vi "Test DAQ IO API.vi"() -> ()   [LabVIEW 2016]
doc: "DAQ IO API Tester."
uses:
  DI Channel Setting.ctl
  DO Channel Setting.ctl
  <vilib>/Utility/miscctls.llb/LVPointTypeDef.ctl
  <vilib>/Utility/error.llb/DialogType.ctl
  DAQ IO.lvlib
panel:
  in  "REQ Retry DI":bool
  in  "REQ Wakeup_helper_loop_DI":bool
  in  "DO Channel Setting":T1
  in  "REQ Acq DI":bool
  in  "DI Channel Setting":T2
  out "Acquire DI":bool[](array[boolean])
  in  "REQ Close DO":bool
  in  "REQ Close DI":bool
  in  "DO Value":bool[](array[boolean])
  in  "REQ Write DO":bool
  out "Connect?":bool
  out "Connect?":bool
  in  "REQ Initialize DO":bool
  in  "DAQ Type":enum16{"Hardware", "Simulation"}(ring)
  in  "REQ Initialize DI":bool
  in  "Show Diagram on Init":bool
  in  "Show Block Diagram":bool
  in  "Stop Module":bool
  in  "Start Module":bool
  in  "Hide Module Panel":bool
  in  "Show Module Panel":bool
  out "Status":string
  out "Module Running?":bool
  # "This VI tests the API for the Module."
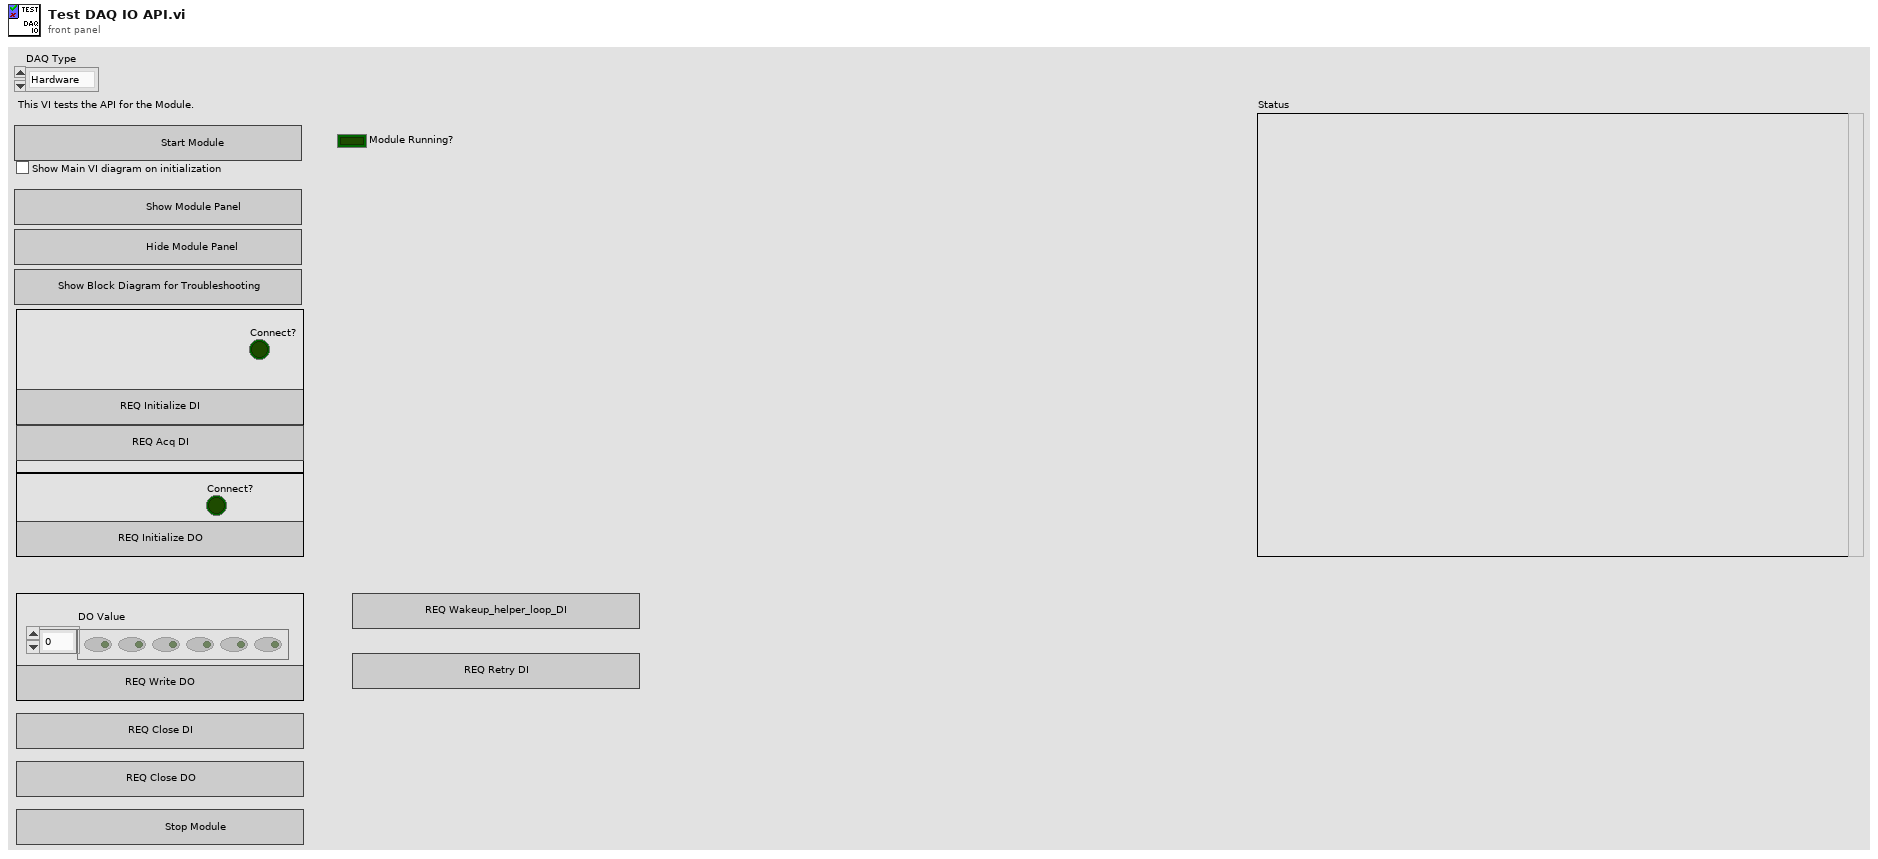
[diagram p1: front panel]
types:
  T1 = typedef "DAQ IO.lvlib/DO Channel Setting.ctl" = cluster{"DO Channel":string[]}
  T2 = typedef "DAQ IO.lvlib/DI Channel Setting.ctl" = cluster{"Channel":string[]}
  T3 = typedef "LVPointTypeDef.ctl" = cluster{"Horizontal":i16, "Vertical":i16}
  T4 = typedef "DAQ IO.lvlib/Broadcast Events--cluster.ctl" = cluster{"Module Did Init":refnum<user-event>, "Status Updated":refnum<user-event>, "Error Reported":refnum<user-event>, "Module Did Stop":refnum<user-event>, "Update Module Execution Status":refnum<user-event>, "REQ Broadcast DI":refnum<user-event>}
  T5 = typedef "DialogType.ctl" = u16
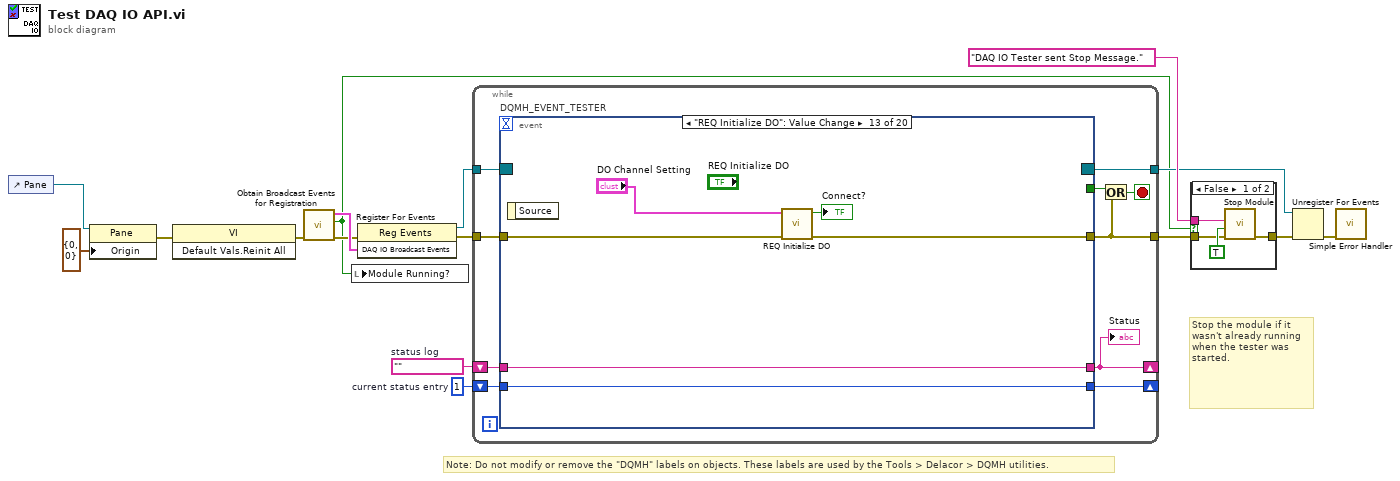
[diagram p0: block diagram]
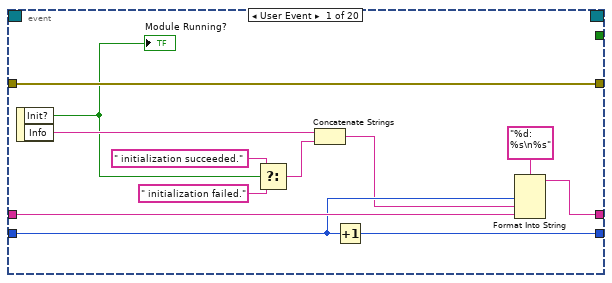
[diagram p3: hidden frame]
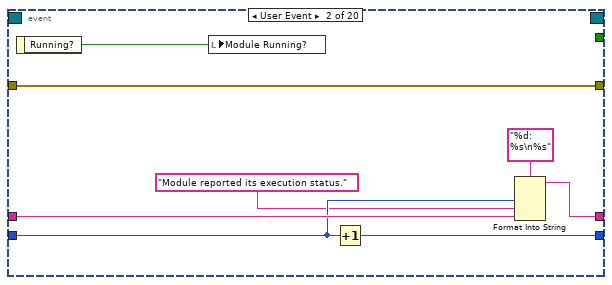
[diagram p4: hidden frame]
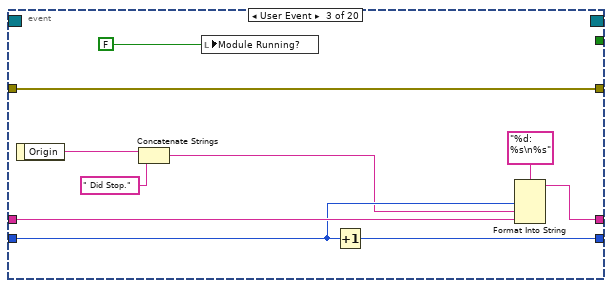
[diagram p5: hidden frame]
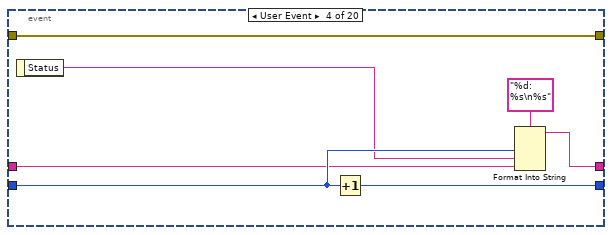
[diagram p6: hidden frame]
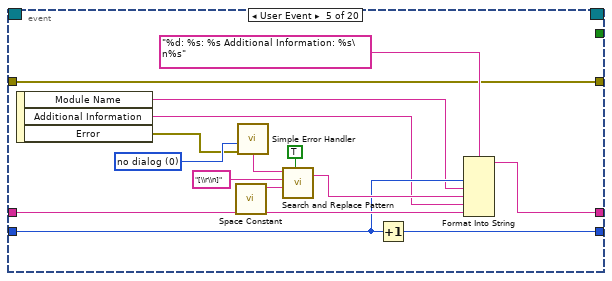
[diagram p7: hidden frame]
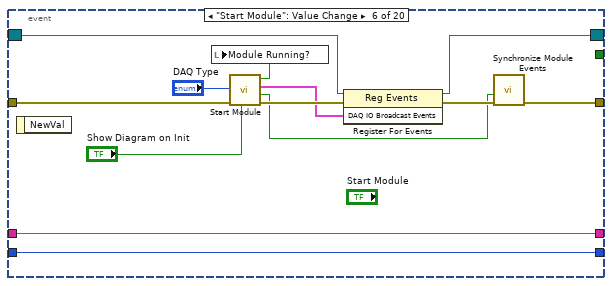
[diagram p8: hidden frame]
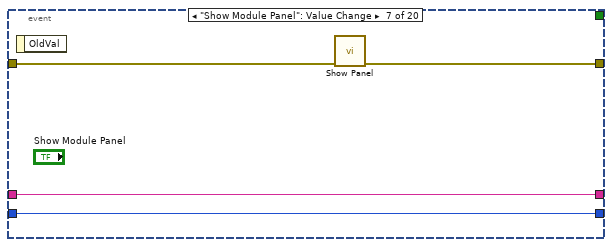
[diagram p9: hidden frame]
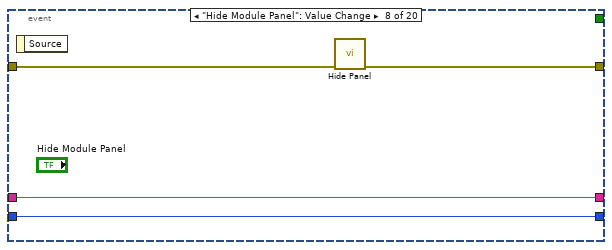
[diagram p10: hidden frame]
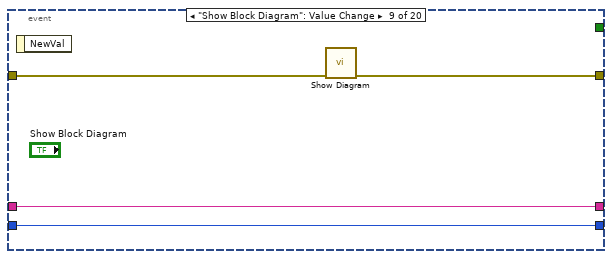
[diagram p11: hidden frame]
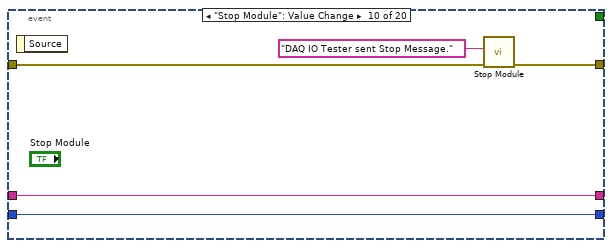
[diagram p12: hidden frame]
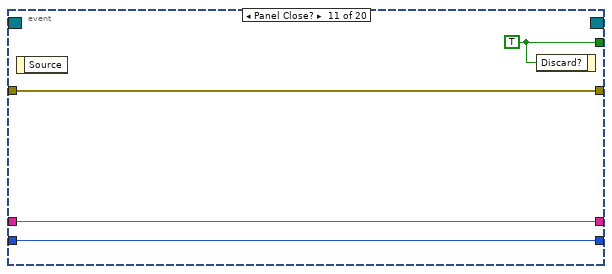
[diagram p13: hidden frame]
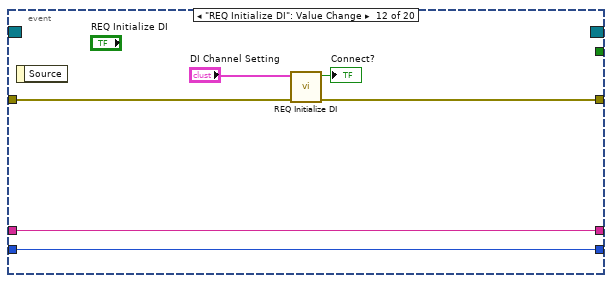
[diagram p14: hidden frame]
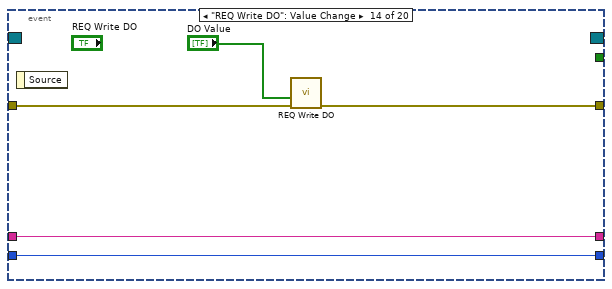
[diagram p15: hidden frame]
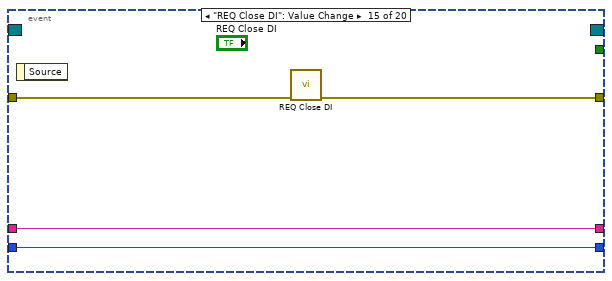
[diagram p16: hidden frame]
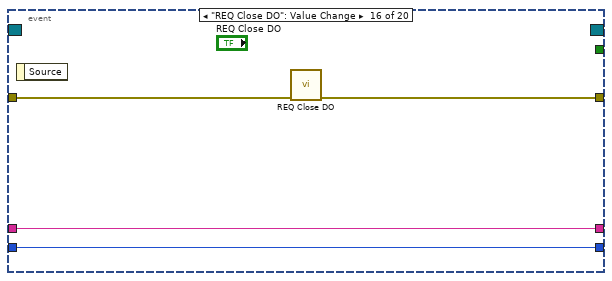
[diagram p17: hidden frame]
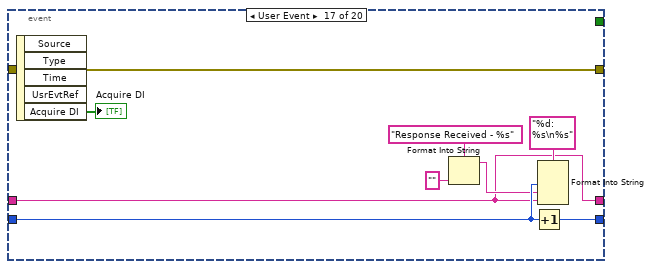
[diagram p18: hidden frame]
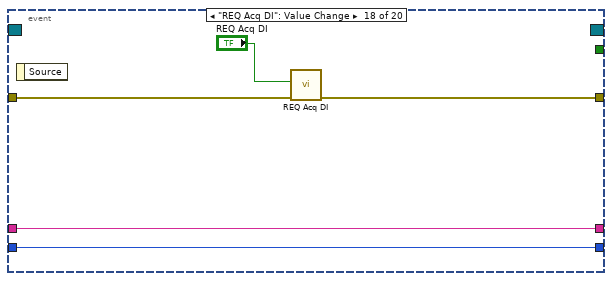
[diagram p19: hidden frame]
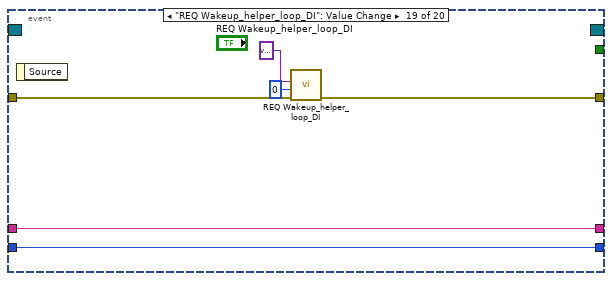
[diagram p20: hidden frame]
diagram:
  w13 = 1  # current status entry
  w14 = ""  # status log
  # "Stop the module if it wasn't already running when the tester was started."
  # "Note: Do not modify or remove the \"DQMH\" labels on objects. These labels are used by the Tools > Delacor > DQMH utilities."
  n1 = control-ref of="Pane"() -> (w1:refnum<vi>)
  n2 = property class="Pane"(reference=w1, "Origin"=T3 {"Horizontal"=0, "Vertical"=0}) -> (error out=w2:errorcluster)  [unwired: 1 in, 1 out]
  n3 = invoke class="VI" method="Default Vals.Reinit All"(error in=w2) -> (error out=w8:errorcluster)  [unwired: 2 in, 2 out]
  n4 = call "Obtain Broadcast Events for Registration.vi"("error in"=w8) -> ("error out"=w7:errorcluster, "Already running?"=w6:bool, "DAQ IO Broadcast Events"=w11:T4)  [unwired: 8 in]
  n5 = local write "Module Running?"(w6) -> ()
  n6 = register-events(error in=w7, w11) -> (reference out=w10:refnum<event-registration>, error out=w12:errorcluster)  [unwired: 1 in]
  n7 = while {
    tunnel: w10 -> [w26]
    tunnel: [w17] -> w5
    shift-right: [w21] -> _
    shift-left: w14 -> [w23]
    shift-right: [w22] -> _
    shift-left: w13 -> [w24]
    tunnel: w12 -> [w19]
    tunnel: [w18] -> w9
    stop <- w20 stop-if-true
    n8 = event "DQMH_EVENT_TESTER" shown="[12] \"REQ Initialize DO\": Value Change" {
      selector: w26 -> [_ _ _ _ _ w85 _ _ _ _ _ _ _ _ _ _ _ _ _ _]
      dyn-events: [_ _ _ _ _ w84 _ _ _ _ _ _ _ _ _ _ _ _ _ _] -> w18
      timeout: _ -> [_ _ _ _ _ _ _ _ _ _ _ _ _ _ _ _ _ _ _ _]
      tunnel: [_ _ _ _ _ _ _ _ _ _ w112 _ _ _ _ _ _ _ _ _] -> w25
      tunnel: [w38 w40 w47 w57 w67 w83 w95 w99 w100 w106 w109 w115 w121 w126 w130 w134 w146 w148 w154 w158] -> w17
      tunnel: w24 -> [w35 w44 w54 w60 w70 w88 w93 w97 w101 w107 w110 w116 w122 w127 w131 w135 w145 w149 w155 w159]
      tunnel: w23 -> [w36 w45 w55 w59 w71 w89 w94 w98 w102 w108 w111 w117 w123 w128 w132 w136 w138 w150 w156 w160]
      tunnel: [w33 w42 w52 w61 w69 w89 w94 w98 w102 w108 w111 w117 w123 w128 w132 w136 w138 w150 w156 w160] -> w21
      tunnel: [w34 w43 w53 w63 w68 w88 w93 w97 w101 w107 w110 w116 w122 w127 w131 w135 w144 w149 w155 w159] -> w22
      tunnel: w19 -> [w38 w40 w47 w57 w67 w82 w92 w96 w103 w104 w109 w118 w124 w129 w133 w137 w146 w151 w157 w161]
      event User Event {
        n9 = event-data() -> ("Init?"=w30:bool, "Info"=w32:string)  [unwired: 1 in]
        "Module Running?" <- w30
        n10 = Select(t=" initialization succeeded.", s=w30, f=" initialization failed.") -> (s? t:f=w27:string)
        n11 = Concatenate Strings(w32, w27) -> (w31:string)
        n12 = Increment(x=w35) -> (x+1=w34:i32)
        n13 = Format Into String(format string="%d: %s\n%s", w35, w31, w36) -> (resulting string=w33:string)  [unwired: 2 in, 1 out]
      }
      event User Event {
        n14 = event-data() -> ("Running?"=w39:bool)  [unwired: 1 in]
        n15 = local write "Module Running?"(w39) -> ()
        n16 = Increment(x=w44) -> (x+1=w43:i32)
        n17 = Format Into String(format string="%d: %s\n%s", w44, "Module reported its execution status.", w45) -> (resulting string=w42:string)  [unwired: 2 in, 1 out]
      }
      event User Event {
        n18 = event-data() -> ("Origin"=w51:string)  [unwired: 1 in]
        n19 = Concatenate Strings(w51, " Did Stop.") -> (w50:string)
        n20 = local write "Module Running?"(FALSE ("Module Did Init?")) -> ()
        n21 = Increment(x=w54) -> (x+1=w53:i32)
        n22 = Format Into String(format string="%d: %s\n%s", w54, w50, w55) -> (resulting string=w52:string)  [unwired: 2 in, 1 out]
      }
      event User Event {
        n23 = event-data() -> ("Status"=w58:string)  [unwired: 1 in]
        n24 = Increment(x=w60) -> (x+1=w63:i32)
        n25 = Format Into String(format string="%d: %s\n%s", w60, w58, w59) -> (resulting string=w61:string)  [unwired: 2 in, 1 out]
      }
      event User Event {
        w72 = T5 0 items=["no dialog", "OK message", "continue or stop message", "OK message + warnings", "continue/stop + warnings"] ("type of dialog (OK msg:1)")
        n26 = event-data() -> ("Module Name"=w66:string, "Additional Information"=w65:string, "Error"=w64:errorcluster)  [unwired: 1 in]
        n27 = call <vilib>:"Space Constant.vi"() -> ("String"=w76:string)
        n28 = call <vilib>:"Simple Error Handler.vi"("type of dialog (OK msg:1)"=w72, "error in (no error)"=w64) -> ("message"=w73:string)  [unwired: 3 in, 4 out]
        n29 = call <vilib>:"Search and Replace Pattern.vi"("string"=w73, "regular expression (\"\")"="[\\r\\n]" ("regular expression (\"\")"), "replace string (\"\")"=w76, "replace all? (F)"=TRUE ("replace all CR/LF with spaces")) -> ("result string"=w74:string)  [unwired: 1 in, 1 out]
        n30 = Increment(x=w70) -> (x+1=w68:i32)
        n31 = Format Into String(format string="%d: %s: %s Additional Information: %s\n%s", w70, w66, w74, w65, w71) -> (resulting string=w69:string)  [unwired: 2 in, 1 out]
      }
      event "Start Module": Value Change {
        n32 = event-data() -> ()  [unwired: 1 in, 1 out]
        n33 = call "Start Module.vi"("Show Main VI Diagram on Init (F)"="Show Diagram on Init", "error in"=w82, "DAQ Type"="DAQ Type") -> ("error out"=w90:errorcluster, "Wait for Event Sync?"=w87:bool, "DAQ IO Broadcast Events"=w86:T4, "Module Was Already Running?"=w81:bool)  [unwired: 5 in]
        n34 = local write "Module Running?"(w81) -> ()
        n35 = register-events(reference=w85, error in=w90, w86) -> (reference out=w84:refnum<event-registration>, error out=w91:errorcluster)
        n36 = call "Synchronize Module Events.vi"("error in"=w91, "Wait for Event Sync?"=w87) -> ("error out"=w83:errorcluster)  [unwired: 9 in]
      }
      event "Show Module Panel": Value Change {
        n37 = event-data() -> ()  [unwired: 1 in, 1 out]
        n38 = call "Show Panel.vi"("error in (no error)"=w92) -> ("error out"=w95:errorcluster)  [unwired: 10 in]
      }
      event "Hide Module Panel": Value Change {
        n39 = event-data() -> ()  [unwired: 1 in, 1 out]
        n40 = call "Hide Panel.vi"("error in (no error)"=w96) -> ("error out"=w99:errorcluster)  [unwired: 10 in]
      }
      event "Show Block Diagram": Value Change {
        n41 = event-data() -> ()  [unwired: 1 in, 1 out]
        n42 = call "Show Diagram.vi"("error in (no error)"=w103) -> ("error out"=w100:errorcluster)  [unwired: 10 in]
      }
      event "Stop Module": Value Change {
        n43 = event-data() -> ()  [unwired: 1 in, 1 out]
        n44 = call "Stop Module.vi"("error in"=w104, "Origin"="DAQ IO Tester sent Stop Message.") -> ("error out"=w106:errorcluster)  [unwired: 9 in]
      }
      event Panel Close? {
        w112 = TRUE ("Discard?")
        n45 = event-data() -> ()  [unwired: 1 in, 1 out]
        n46 = event-data("Discard?"=w112) -> ()  [unwired: 1 in, 1 out]
      }
      event "REQ Initialize DI": Value Change {
        n47 = event-data() -> ()  [unwired: 1 in, 1 out]
        n48 = call "REQ Initialize DI.vi"("error in"=w118, "DI Channel Setting"="DI Channel Setting") -> ("error out"=w115:errorcluster, "Connect?"=→"Connect?":bool)  [unwired: 7 in, 1 out]
      }
      event "REQ Initialize DO": Value Change {
        n49 = event-data() -> ()  [unwired: 1 in, 1 out]
        n50 = call "REQ Initialize DO.vi"("error in"=w124, "DO Channel Setting"="DO Channel Setting") -> ("error out"=w121:errorcluster, "Connect?"=→"Connect?":bool)  [unwired: 7 in, 1 out]
      }
      event "REQ Write DO": Value Change {
        n51 = event-data() -> ()  [unwired: 1 in, 1 out]
        n52 = call "REQ Write DO.vi"("error in"=w129, "DO Value"="DO Value") -> ("error out"=w126:errorcluster)  [unwired: 9 in]
      }
      event "REQ Close DI": Value Change {
        n53 = event-data() -> ()  [unwired: 1 in, 1 out]
        n54 = call "REQ Close DI.vi"("error in"=w133) -> ("error out"=w130:errorcluster)  [unwired: 10 in]
      }
      event "REQ Close DO": Value Change {
        n55 = event-data() -> ()  [unwired: 1 in, 1 out]
        n56 = call "REQ Close DO.vi"("error in"=w137) -> ("error out"=w134:errorcluster)  [unwired: 10 in]
      }
      event User Event {
        n57 = event-data() -> ("Acquire DI"=→"Acquire DI":bool[])  [unwired: 1 in, 4 out]
        n58 = Format Into String(format string="Response Received - %s", "" ("input 1")) -> (resulting string=w141:string)  [unwired: 2 in, 1 out]
        n59 = Increment(x=w145) -> (x+1=w144:i32)
        n60 = Format Into String(format string="%d: %s\n%s", w145, w141, w138) -> ()  [unwired: 2 in, 2 out]
      }
      event "REQ Acq DI": Value Change {
        n61 = event-data() -> ()  [unwired: 1 in, 1 out]
        n62 = call "REQ Acq DI.vi"("error in"=w151, "Acq DI"="REQ Acq DI") -> ("error out"=w148:errorcluster)  [unwired: 9 in]
      }
      event "REQ Wakeup_helper_loop_DI": Value Change {
        n63 = event-data() -> ()  [unwired: 1 in, 1 out]
        n64 = call "REQ Wakeup_helper_loop_DI.vi"("error in"=w157, "Timeout"=0, "Data"=variant) -> ("error out"=w154:errorcluster)  [unwired: 8 in]
      }
      event "REQ Retry DI": Value Change {
        n65 = event-data() -> ()  [unwired: 1 in, 1 out]
        n66 = call "REQ Retry DI.vi"("error in"=w161) -> ("error out"=w158:errorcluster)  [unwired: 10 in]
      }
    }
    "Status" <- w21
    n67 = Or(x=w25, y=w17) -> (x .or. y?=w20:bool)
  }
  n68 = case shown="False" w6 {
    tunnel: [w165 w166] -> w16
    tunnel: "DAQ IO Tester sent Stop Message." ("Origin") -> [w164 _]
    tunnel: w5 -> [w162 w166]
    frame False {
      n69 = call "Stop Module.vi"("error in"=w162, "Wait for Module to Stop? (F)"=TRUE ("Wait for Module to stop?"), "Origin"=w164) -> ("error out"=w165:errorcluster)  [unwired: 8 in]
    }
    frame True {
    }
  }
  n70 = Unregister For Events(event registration refnum=w9, error in=w16) -> (error out=w4:errorcluster)
  n71 = call <vilib>:"Simple Error Handler.vi"("error in (no error)"=w4) -> ()  [unwired: 4 in, 5 out]
